vi "rearrangeClusterElements.vi"(8 "error in (no error)":errorcluster, 11 "TypeConstructor in":refnum<class "TypeConstructor.lvclass">) -> (0 "error out":errorcluster, 3 "TypeConstructor out":refnum<class "TypeConstructor.lvclass">)   [LabVIEW 2012, in "TypeConstructor.lvclass"]
uses:
  TypeConstructor.lvclass
  TypeConstructor.lvclass/TypeConstructor.ctl
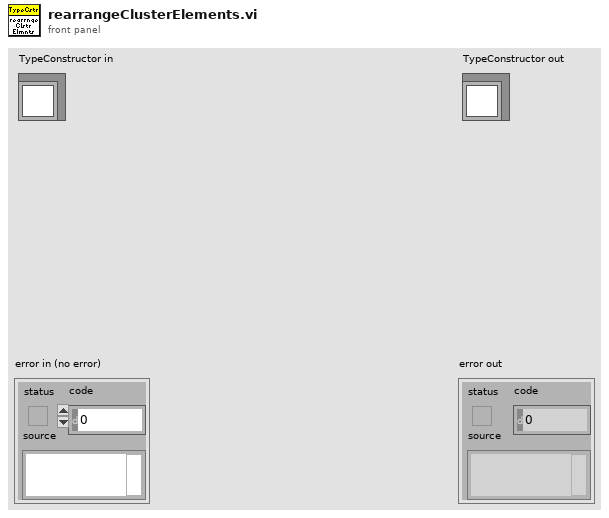
[diagram p1: front panel]
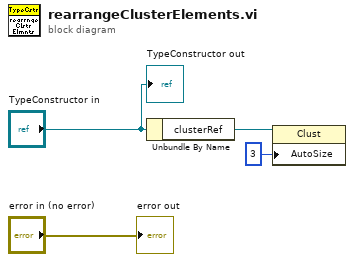
[diagram p0: block diagram]
diagram:
  n1 = Unbundle By Name("TypeConstructor in") -> ("clusterRef"=w2:refnum<vi>)
  n2 = property class="Clust"(reference=w2, "AutoSize"=u32 3 ("Auto Sizing")) -> ()  [unwired: 1 in, 2 out]
  "error out" <- "error in (no error)"
  "TypeConstructor out" <- "TypeConstructor in"
